vi "Part 2.vi"(11 "Input":string) -> (3 "Output":i64)   [LabVIEW 2021]
uses:
  d1da3a3e-bfd9-4d7e-ab5d-c040725d0ddb.vi
  1f8f5492-5d10-49a7-ba1f-8a21850da122.vi
  <userlib>/_OpenG.lib/array/array.llb/Search 1D Array (String)__ogtk.vi
  <userlib>/_OpenG.lib/array/array.llb/Index 1D Array Elements (String)__ogtk.vi
  <userlib>/_OpenG.lib/array/array.llb/Search 1D Array (Boolean)__ogtk.vi
panel:
  out "map in":map{string, string[]}(c390)
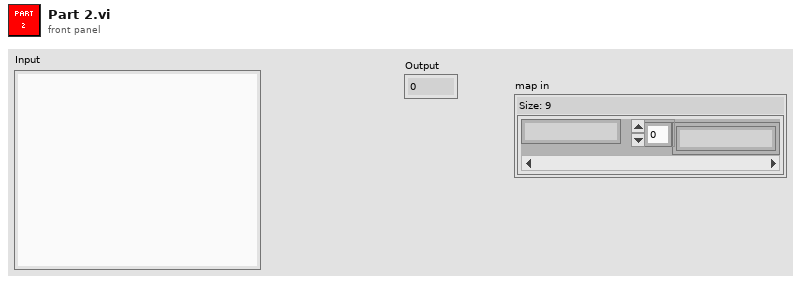
[diagram p1: front panel]
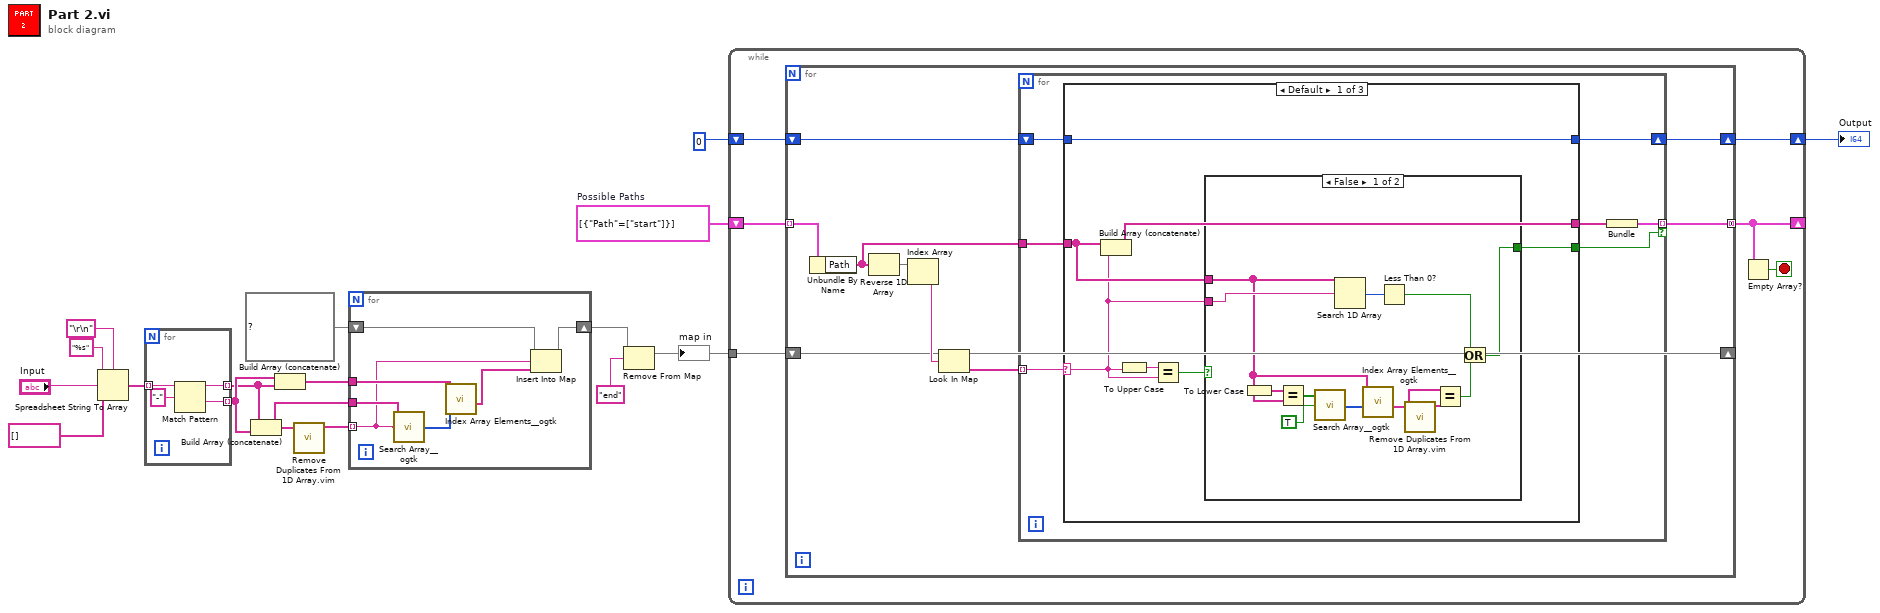
[diagram p0: block diagram]
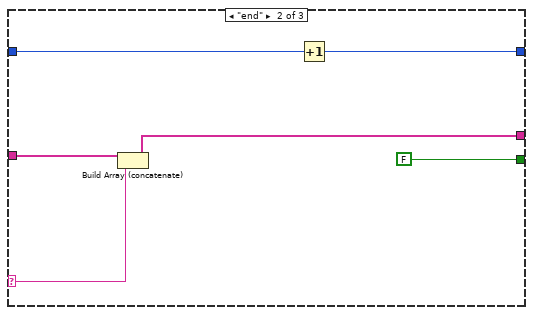
[diagram p3: hidden frame]
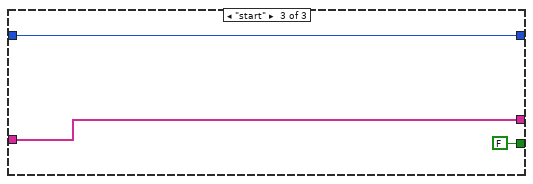
[diagram p4: hidden frame]
diagram:
  w5 = cluster{"Path":string[]}[] [{"Path"=["start"]}]  # Possible Paths
  n1 = Spreadsheet String To Array(delimiter (Tab)="\r\n", format string="%s", spreadsheet string="Input", array type (2D Dbl)=string[] []) -> (array=w14:string[])
  n2 = for {
    tunnel: w14 -> [w21] mode=indexing
    tunnel: [w19] -> w11 mode=indexing
    tunnel: [w18] -> w12 mode=indexing
    n3 = Match Pattern(string=w21, regular expression="-") -> (before substring=w19:string, after substring=w18:string)  [unwired: 1 in, 2 out]
  }
  n4 = Build Array (concatenate)(w11, w12) -> (w10:string[])
  n5 = Build Array (concatenate)(w12, w11) -> (w9:string[])
  n6 = call "Remove Duplicates From 1D Array.vim"("array"=w10) -> ("array with duplicates removed"=w13:string[])  [unwired: 10 in]
  n7 = for {
    tunnel: w13 -> [w25] mode=indexing
    tunnel: w10 -> [w28]
    tunnel: w9 -> [w27]
    shift-right: [w22] -> w7
    shift-left: map{string, string[]} {} ("map in") -> [w23]
    n8 = call-poly <userlib>:"Search Array__ogtk.vi"("Array"=w28, "Element Data"=w25) -> ("Indices of Elements"=w26:i32[])  [unwired: 7 in]
    n9 = call-poly <userlib>:"Index Array Elements__ogtk.vi"("indices"=w26, "array"=w27) -> ("elements"=w24:string[])  [unwired: 9 in]
    n10 = Insert Into Map(map in=w23, key=w25, value=w24) -> (map out=w22:map{string, string[]})  [unwired: 2 out]
  }
  n11 = Remove From Map(10:"end" ("key"), 11:w7) -> (3:w3:map{string, string[]})  [unwired: 2 out]
  "map in" <- w3
  n12 = while {
    shift-right: [w29] -> _
    shift-left: w5 -> [w33]
    shift-right: [w31] -> w1
    shift-left: i64 0 -> [w32]
    tunnel: w3 -> [w30]
    stop <- w34 stop-if-true
    n13 = for {
      tunnel: w33 -> [w36] mode=indexing
      shift-right: [w39] -> w31
      shift-left: w32 -> [w40]
      shift-right: [w41] -> _
      shift-left: w30 -> [w41]
      tunnel: [w35] -> w29 mode=concatenating
      n14 = Unbundle By Name(w36) -> ("Path"=w37:string[])
      n15 = Reverse 1D Array(array=w37) -> (reversed array=w43:string[])
      n16 = Index Array(array=w43) -> (element=w42:string)  [unwired: 1 in]
      n17 = Look In Map(map=w41, key=w42) -> (value=w38:string[])  [unwired: 1 in, 1 out]
      n18 = for {
        shift-right: [w48] -> w39
        shift-left: w40 -> [w49]
        tunnel: w38 -> [w50] mode=indexing
        tunnel: w37 -> [w46]
        tunnel: [w44] -> w35 mode=indexing if=w47
        n19 = case shown="Default" w50 {
          selector: w50 -> [w51 w72 _]
          tunnel: w49 -> [w57 w76 w79]
          tunnel: [w57 w75 w79] -> w48
          tunnel: [w53 FALSE FALSE] -> w47
          tunnel: w46 -> [w52 w73 w77]
          tunnel: [w56 w71 w77] -> w45
          frame Default {
            n20 = Build Array (concatenate)(w52, w51) -> (w56:string[])
            n21 = To Upper Case(1:w51) -> (0:w55:string)
            n22 = Equal?(x=w55, y=w51) -> (x = y?=w54:bool)
            n23 = case shown="False" w54 {
              selector: w54 -> [_ w70]
              tunnel: [w59 w70] -> w53
              tunnel: w52 -> [w62 _]
              tunnel: w51 -> [w69 _]
              frame False {
                n24 = To Lower Case(string=w62) -> (all lower case string=w67:string[])
                n25 = Equal?(x=w67, y=w62) -> (x = y?=w66:bool[])
                n26 = call-poly <userlib>:"Search Array__ogtk.vi"("Array"=w66, "Element Data"=TRUE) -> ("Indices of Elements"=w64:i32[])  [unwired: 7 in]
                n27 = Search 1D Array(1D array=w62, element=w69) -> (index of element=w68:i32)  [unwired: 1 in]
                n28 = call-poly <userlib>:"Index Array Elements__ogtk.vi"("indices"=w64, "array"=w62) -> ("elements"=w58:string[])  [unwired: 9 in]
                n29 = Less Than 0?(x=w68) -> (x < 0?=w60:bool)
                n30 = call "Remove Duplicates From 1D Array.vim"("array"=w58) -> ("array with duplicates removed"=w63:string[])  [unwired: 10 in]
                n31 = Equal?(x=w58, y=w63) -> (x = y?=w61:bool)
                n32 = Or(x=w60, y=w61) -> (x .or. y?=w59:bool)
              }
              frame True {
              }
            }
          }
          frame "end" {
            n33 = Build Array (concatenate)(w73, w72) -> (w71:string[])
            n34 = Increment(x=w76) -> (x+1=w75:i64)
          }
          frame "start" {
          }
        }
        n35 = Bundle("Path"=w45) -> (w44:cluster{"Path":string[]})  [unwired: 1 in]
      }
    }
    n36 = Empty Array?(array=w29) -> (empty?=w34:bool)
  }
  "Output" <- w1
